vi "PH_BeamlineController.set Source GUI Elements.vi"(0 "VI in":refnum<vi>, 5 "error in (no error)":errorcluster) -> (14 "VI out":refnum<vi>, 19 "error out":errorcluster)   [LabVIEW 2014, in "PH_BeamlineController.lvlib"]
uses:
  PH_BeamlineController.lvlib
  PH_Basics/PH_SystemInformation/PH_SystemInformationEnabling State.ctl
  PH_Basics/PH_SystemInformation/PH_SystemInformation.lvlib
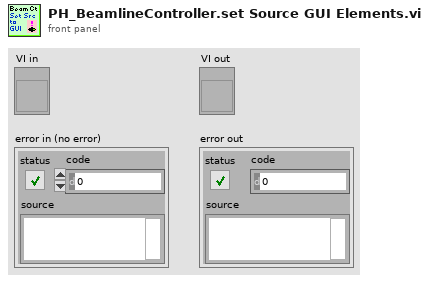
[diagram p1: front panel]
types:
  T1 = enum8{"Enabled", "Disabled", "Disabled and Grayed Out"}
  T2 = typedef "PH_SystemInformation.lvlib/PH_SystemInformationEnabling State.ctl" = i32
  T3 = enum16{"Laser", "PreAmp", "MainAmp", "Exp 1", "Exp 2", "Exp 3", "Exp 4"}
  T4 = typedef "PH_BeamlineController.lvlib/PH_BeamlineController.i attribute.ctl" = cluster{"Vacuum Exp LB":cluster{"Channel":string, "Limit [mbar]":dbl, "Pressure [mbar]":dbl, "GUI Ref":refnum<vi>}, "Sources":T5[], "PA DP Targets":T7[], "Path":cluster{"Source":T6, "PA DP Target":T8, "Target":T9}, "Targets":cluster{"Name":T9, "GUI Ref":refnum<vi>, "Current State":bool, "Wanted State":bool, "Enabled":bool}[], "Status Tags":cluster{"Name":string, "Status":T10}[], "special GUI Refs":T11}
  T5 = typedef "PH_BeamlineController.lvlib/PH_BeamlineController.Source Attributes.ctl" = cluster{"Name":T6, "GUI Ref":refnum<vi>, "Current State":bool, "Wanted State":bool}
  T6 = typedef "PH_BeamlineController.lvlib/PH_BeamlineController.Sources.ctl" = enum16{"None", "YLF", "fs-Frontend", "ns-Frontend", "YLF and ns-Frontend", "fs- and ns-Frontend"}
  T7 = typedef "PH_BeamlineController.lvlib/PH_BeamlineController.PA DP Target Attributes.ctl" = cluster{"Name":T8, "GUI Ref":refnum<vi>, "Current State":bool, "Wanted State":bool, "Enabled":bool}
  T8 = typedef "PH_BeamlineController.lvlib/PH_BeamlineController.PA DP Targets.ctl" = enum16{"None", "Dump PA Delayed Beam", "Dump PA Undelayed Beam", "Dumps PA Delayed and Undelayed Beam"}
  T9 = typedef "PH_BeamlineController.lvlib/PH_BeamlineController.Targets.ctl" = enum16{"None", "PreAmp", "Dump Exp Laserlab", "Exp Laserlab", "Calorimeter", "Dump Exp Laserbay", "Exp Laserbay", "Dump Exp Z6", "Exp Z6"}
  T10 = typedef "PH_StatusHandler.lvlib/PH_StatusHandler.Status.ctl" = i16
  T11 = typedef "PH_BeamlineController.lvlib/PH_BeamlineController.special GUI Refs.ctl" = cluster{"PA-Backreflection-Meas":refnum<vi>, "fs_Synchrolock_Watch":refnum<vi>}
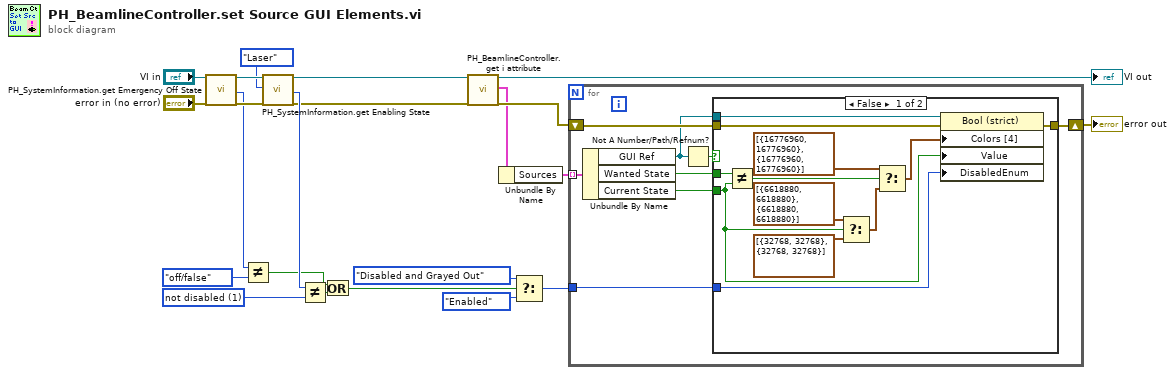
[diagram p0: block diagram]
diagram:
  w12 = T2 1 items=["no info", "not disabled", "disabled"] ("y")
  n1 = call "PH_SystemInformation.get Emergency Off State.vi"("i ref in"="VI in", "error in (no error)"="error in (no error)") -> ("i ref out"=w18:refnum<vi>, "Emergency Off State"=w15:enum16{"no info", "off/false", "Alarm"}, "error out"=w17:errorcluster)  [unwired: 15 in]
  n2 = Not Equal?(x=w15, y=enum16{"no info", "off/false", "Alarm"}."off/false") -> (x != y?=w11:bool)
  n3 = call "PH_SystemInformation.get Enabling State.vi"("i ref in"=w18, "Wanted State"=T3."Laser", "error in (no error)"=w17) -> ("i ref out"=w8:refnum<vi>, "Enabling State"=w13:T2, "error out"=w6:errorcluster)  [unwired: 14 in]
  n4 = Not Equal?(x=w13, y=w12) -> (x != y?=w10:bool)
  n5 = Or(x=w11, y=w10) -> (x .or. y?=w5:bool)
  n6 = call "PH_BeamlineController.get i attribute.vi"("i ref in"=w8, "error in (no error)"=w6) -> ("i ref out"=→"VI out":refnum<vi>, "i attribute"=w19:T4, "error out"=w21:errorcluster)  [unwired: 15 in]
  n7 = Unbundle By Name(w19) -> ("Sources"=w1:T5[])
  n8 = Select(t=T1."Disabled and Grayed Out" ("Disabled"), s=w5, f=T1."Enabled" ("Disabled")) -> (s? t:f=w2:T1)
  n9 = for {
    shift-right: [w29] -> w20
    shift-left: w21 -> [w30]
    tunnel: w1 -> [w28] mode=indexing
    tunnel: w2 -> [w23]
    n10 = Unbundle By Name(w28) -> ("GUI Ref"=w25:refnum<vi>, "Wanted State"=w27:bool, "Current State"=w26:bool)
    n11 = Not A Number/Path/Refnum?(number/path/refnum=w25) -> (NaN/Path/Refnum?=w24:bool)
    n12 = case shown="False" w24 {
      tunnel: w30 -> [w42 w43]
      tunnel: [w41 w43] -> w29
      tunnel: w25 -> [w40 _]
      tunnel: w27 -> [w35 _]
      tunnel: w26 -> [w34 _]
      tunnel: w23 -> [w33 _]
      frame False {
        n13 = Not Equal?(x=w35, y=w34) -> (x != y?=w38:bool)
        n14 = Select(t=cluster{"Color Box":u32, "Color Box 2":u32}[] [{"Color Box"=6618880, "Color Box 2"=6618880}, {"Color Box"=6618880, "Color Box 2"=6618880}], s=w34, f=cluster{"Color Box":u32, "Color Box 2":u32}[] [{"Color Box"=32768, "Color Box 2"=32768}, {"Color Box"=32768, "Color Box 2"=32768}]) -> (s? t:f=w36:cluster{"Color Box":u32, "Color Box 2":u32}[])
        n15 = Select(t=cluster{"Color Box":u32, "Color Box 2":u32}[] [{"Color Box"=16776960, "Color Box 2"=16776960}, {"Color Box"=16776960, "Color Box 2"=16776960}], s=w38, f=w36) -> (s? t:f=w37:cluster{"Color Box":u32, "Color Box 2":u32}[])
        n16 = property class="Bool (strict)"(reference=w40, error in=w42, "Colors [4]"=w37, "Value"=w34, "DisabledEnum"=w33) -> (error out=w41:errorcluster)  [unwired: 1 out]
      }
      frame True {
      }
    }
  }
  "error out" <- w20
